vi "Write Digitizer Channel.vi"(8 "error in (no error)":errorcluster, 10 "Digitizer Channel Setting":T1={"Max"=10.0, "Min"=0.0, "Data Reduction"="None", "Averging Points"=1000, "Decimate Interval"=0, "Aperture Options"={"Tolerance"=0, "Burst"=0, "Min SampleRate"=1000, "Min SampleIndex"=0}} {"Decimate Interval" format="%.0p"; "Averging Points" format="%.0p"; "Aperture Options"."Min SampleIndex" format="%.0p"; "Aperture Options"."Min SampleRate" format="%.0p"}, 11 "Digitizer Channel configuration":refnum<class "Digitizer Channel configuration.lvclass">) -> (0 "error out":errorcluster, 3 "Digitizer Channel configuration out":refnum<class "Digitizer Channel configuration.lvclass">)   [LabVIEW 2025, in "Digitizer.lvlib" / "Digitizer Channel configuration.lvclass"]
uses:
  Digitizer Channel configuration.lvclass
  Digitizer Channel Setting.ctl
  Digitizer Channel configuration.lvclass/Digitizer Channel configuration.ctl
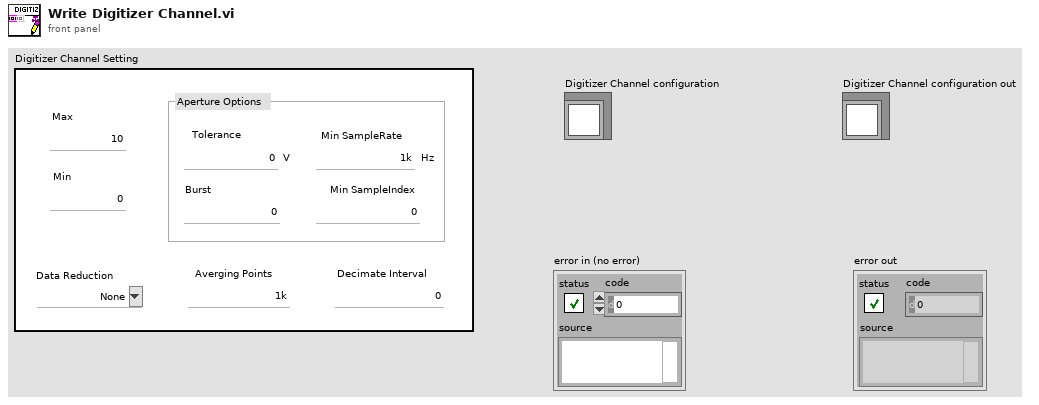
[diagram p1: front panel]
types:
  T1 = typedef "Digitizer.lvlib/Digitizer Channel configuration.lvclass/Digitizer Channel Setting.ctl" = cluster{"Max":dbl, "Min":dbl, "Data Reduction":string, "Averging Points":u32, "Decimate Interval":u32, "Aperture Options":cluster{"Tolerance":u32, "Burst":u32, "Min SampleRate":u32, "Min SampleIndex":u32}}
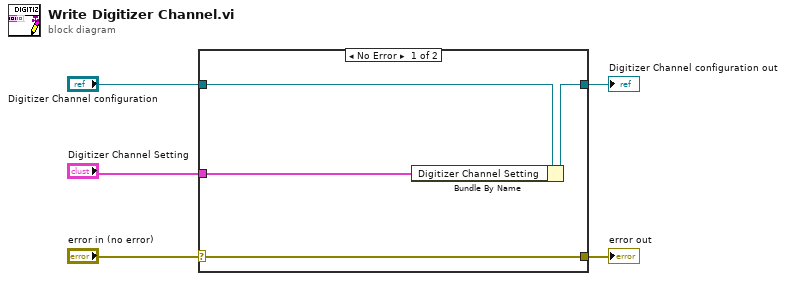
[diagram p0: block diagram]
diagram:
  n1 = case shown="No Error" "error in (no error)" {
    selector: "error in (no error)" -> [w9 w10]
    tunnel: [w9 w10] -> w4
    tunnel: [w7 w11] -> w2
    tunnel: "Digitizer Channel configuration" -> [w8 w11]
    tunnel: "Digitizer Channel Setting" -> [w6 _]
    frame No Error {
      n2 = Bundle By Name(cluster=w8, "Digitizer Channel Setting"=w6) -> (w7:refnum<class "Digitizer Channel configuration.lvclass">)
    }
    frame Error {
    }
  }
  "error out" <- w4
  "Digitizer Channel configuration out" <- w2
